vi "temp limits.vi.vi"(6 "MinTemp (0)":dbl, 7 "MaxTemp (25)":dbl=25.0, 8 "error in (no error)":errorcluster, 10 "TEMP":dbl) -> (0 "error out":errorcluster, 2 "Warning":bool, 3 "Warning Text":string)   [LabVIEW 2014]
doc: "SubVI porównuje temperaturę\nprocesową z zadanymi wartościami granicznymi"
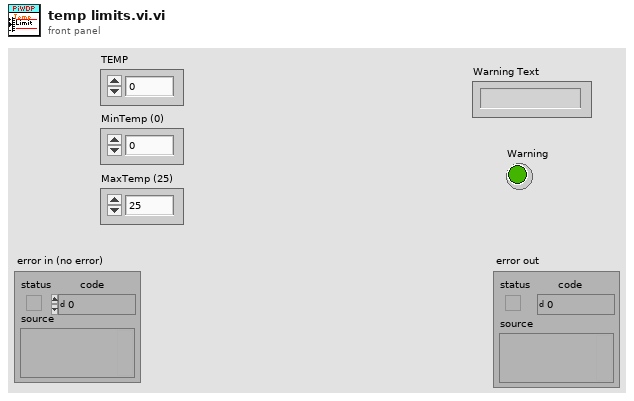
[diagram p1: front panel]
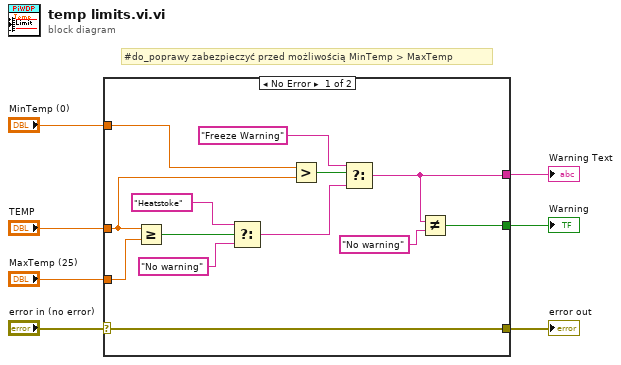
[diagram p0: block diagram]
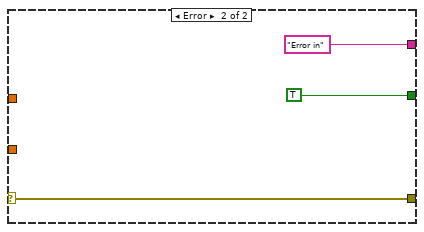
[diagram p2: hidden frame]
diagram:
  # "#do_poprawy zabezpieczyć przed możliwością MinTemp > MaxTemp"
  n1 = case shown="No Error" "error in (no error)" {
    selector: "error in (no error)" -> [w8 w23]
    tunnel: [w8 w23] -> w6
    tunnel: "TEMP" -> [w16 _]
    tunnel: "MinTemp (0)" -> [w15 _]
    tunnel: "MaxTemp (25)" -> [w20 _]
    tunnel: [w11 "Error in"] -> w2
    tunnel: [w9 TRUE] -> w1
    frame No Error {
      n2 = Greater Or Equal?(x=w16, y=w20) -> (x >= y?=w19:bool)
      n3 = Select(t="Heatstoke", s=w19, f="No warning") -> (s? t:f=w13:string)
      n4 = Greater?(x=w15, y=w16) -> (0:w14:bool)
      n5 = Select(t="Freeze Warning", s=w14, f=w13) -> (s? t:f=w11:string)
      n6 = Not Equal?(x=w11, y="No warning") -> (x != y?=w9:bool)
    }
    frame Error {
    }
  }
  "error out" <- w6
  "Warning Text" <- w2
  "Warning" <- w1
